vi "imp_test_v6.vi"() -> ()   [LabVIEW 2014]
uses:
  <vilib>/LabVIEW Targets/FPGA/cRIO/shared/nicrio_ModuleControls/nicrio_cRIO-9237_DataRatesRing.ctl
  <vilib>/LabVIEW Targets/FPGA/cRIO/shared/nicrio_ModuleControls/nicrio_cRIO-9237_ExcitationVoltageRing.ctl
  <vilib>/rvi/FXPMathLib/FxpSinAndCos/subVIs/nifxpmath_SinAndCos_SimConfig.ctl
  <vilib>/rvi/Emulation/niFpgaGetClockAttributes.vi
  <vilib>/rvi/Emulation/niFpgaSctlEmulationGetInTimedLoop.vi
  <vilib>/rvi/Emulation/niFpgaEmulationReportErrorSimple.vi
  <vilib>/rvi/Emulation/niFpgaProcessEmulError.vi
  <vilib>/rvi/interface/RandomDataEmulation/nirviRandomDataMultiElementFPGAFIFO.vi
  <instcachedir>/0/nirviRandomDataMultiElementFPGAFIFO_AD0CFC12EF974623A9C2E4184BC062B2.lvgen/nirviRandomDataMultiElementFPGAFIFO_AD0CFC12EF974623A9C2E4184BC062B2_025.vi
  <vilib>/rvi/interface/RandomDataEmulation/niFpgaRandomDataHandleErrors.vi
  <vilib>/rvi/Emulation/niFpgaCriticalErrorInLSC.vi
  <vilib>/rvi/eio/common/nirviEmuTemplateMethod_errors.vi
  <vilib>/rvi/FXPMathLib/FxpSinAndCos/simVIs/DllFxpSinAndCosTemp_sub.vi
  <vilib>/rvi/eio/common/nirviEmuTemplatePropertySet_errors.vi
  <vilib>/rvi/DataTransferAndStorage/Container/XNode/niFpgaContainer.xnode
  <vilib>/rvi/interface/RandomDataEmulation/nirviRandomDataFpgaMultiElementTemplate.vi
  <vilib>/eio/EIONode/EIONode.xnode
  <vilib>/rvi/FXPMathLib/FxpMul/XNode/nifxpmath_Multiplier.xnode
  <vilib>/rvi/FXPMathLib/FxpSinAndCos/XNode/nifxpmath_SinAndCos.xnode
  <vilib>/rvi/Analysis/measure/butterworth/XNode/niFpgaButterworthFilter.xnode
  <vilib>/rvi/FXPMathLib/FxpSub/XNode/nifxpmath_Sub.xnode
  <vilib>/rvi/FXPMathLib/FxpAdd/XNode/nifxpmath_Add.xnode
  <vilib>/eio/EIOPropertyNode/EIOPropertyNode.xnode
  <vilib>/rvi/eio/common/nirviEmuTemplatePropertyGet_errors.vi
  <vilib>/rvi/eio/common/nirviEmuTemplatePropertyGet_noerrors.vi
  <vilib>/rvi/eio/common/nirviEmuTemplatePropertySet_noerrors.vi
  <vilib>/rvi/FXPMathLib/sim/FxpSim.dll
panel:
  out "Strain_y (Avg2 w. f)":fxp<+/-,34,7>
  in  "Strain_y Avg2 coeff.":i32[](array[numeric])=[946630756, 63555534]
  out "Strain_y (Avg4 w. f)":fxp<+/-,35,7>
  in  "Strain_y Avg4 coeff.":i32[](array[numeric])=[946630756, 63555534]
  out "Strain_y (Avg2)":fxp<+/-,30,3>
  out "Strain_y (Avg4)":fxp<+/-,31,3>
  in  "Belt_op":fxp<+/-,7,7>
  in  "Belt_mp":fxp<+/-,6,6>
  in  "Belt_oy":fxp<+/-,7,7>
  in  "Belt_my":fxp<+/-,6,6>
  out "Fp_dc":fxp<+/-,32,10>
  out "Fy_dc":fxp<+/-,32,10>
  in  "Zero_y":bool
  in  "Zero_p":bool
  in  "mt0_omega_p":u32
  in  "Encoder reset":bool
  out "fpt_d":fxp<+/-,36,18>
  out "Dp_error_dd":fxp<+/-,36,16>
  out "Dp_error_d":fxp<+/-,33,8>
  in  "Dp_dd coeff.":i32[](array[numeric])=[946630756, 63555534]
  out "Dp_dd":fxp<+/-,36,25>
  out "dFp_PID":fxp<+/-,36,18>
  in  "dFp_PID coeff.":i32[](array[numeric])=[946630756, 63555534]
  out "fpt_i":fxp<+/-,34,18>
  in  "Bv_p":fxp<+/-,22,8>
  in  "Kv_p":fxp<+/-,22,8>
  out "Dp_error":fxp<+/-,22,7>
  out "Dpr_sin":fxp<+/-,22,7>
  in  "Sin offset_p":fxp<+/-,22,7>
  in  "Sin magnitude_p":fxp<+/-,21,6>
  out "Dpr_sin_dd":fxp<+/-,35,20>
  out "Dpr_sin_d":fxp<+/-,33,15>
  out "Sin omega_p":fxp<+/-,34,9>
  in  "Sin wave freq._p (Hz)":fxp<+/-,32,6>
  in  "Dpr_step":fxp<+/-,22,7>
  out "Dpr_for":fxp<+/-,22,7>
  in  "Command_p":i16(ring) items=["Step", "Sine"]
  in  "Ki_p":fxp<+/-,36,9>
  out "Fp_PID":fxp<+/-,36,16>
  in  "fp_tolorance":fxp<+,22,6>
  out "fp_tilde":fxp<+/-,33,10>
  in  "Kd_p":fxp<+/-,36,9>
  in  "Kp_p":fxp<+/-,36,9>
  out "Fr_p":fxp<+/-,32,10>
  in  "S/F coeff_p":fxp<+/-,25,-10>
  in  "S/F coeff_y":fxp<+/-,25,-10>
  out "va_p":fxp<+/-,36,7>
  out "vb_p":fxp<+/-,37,8>
  out "vq_p_F":fxp<+/-,20,5> format="%.57g"
  out "vd_p_F":fxp<+/-,20,5>
  in  "dFp_add":bool
  in  "Stop motor_p":bool
  out "Force_p":fxp<+/-,32,10>
  in  "Strain selection_p":i16(ring) items=["Raw", "Avg.8", "Avg.8 w. filter"]
  out "Strain_p (Avg8 w. f)":fxp<+/-,36,8>
  in  "Strain_p Avg.8 coeff.":i32[](array[numeric])=[946630756, 63555534]
  out "Strain_p (Avg8)":fxp<+/-,36,4>
  out "Raw Strain_p":fxp<+/-,36,4>
  out "Mod6/AI3":fxp<+/-,36,4>
  in  "Strain gage reset_p":bool
  out "Dp_d (mm/s)":fxp<+/-,36,11>
  out "omega_p (rad/s)":fxp<+/-,20,9>
  out "mt_omega_p":u32
  out "rad_p(NrTheta)":fxp<+/-,33,20>
  out "D_p(mm)":fxp<+/-,32,7>
  out "Encoder Position_p":i32
  in  "Encoder reset_p":bool
  out "Strain_y (Avg8 w. f)":fxp<+/-,36,8>
  in  "Strain_y Avg8 coeff.":i32[](array[numeric])=[-898916953, 1957103773, 3888751]
  out "Dyr_for":fxp<+/-,22,7>
  in  "Command_y":i16(ring) items=["Step", "Sine"]
  out "Strain_y (Avg8)":fxp<+/-,36,4>
  in  "Strain selection_y":i16(ring) items=["Raw", "Avg.8", "Avg.8 w. filter", "Avg.4", "Avg.4 w. filter", "Avg.2", "Avg.2 w. filter"]
  out "vb_y":fxp<+/-,38,8>
  out "va_y":fxp<+/-,38,8>
  out "fyt_d":fxp<+/-,36,18>
  out "Fr_y":fxp<+/-,32,10>
  in  "Bv_y":fxp<+/-,22,8>
  out "Dy_error_dd":fxp<+/-,36,16>
  out "Dy_error_d":fxp<+/-,33,8>
  in  "Kv_y":fxp<+/-,22,8>
  out "Dy_error":fxp<+/-,22,7>
  out "Dyr_sin_dd":fxp<+/-,35,20>
  out "Dyr_sin_d":fxp<+/-,33,15>
  out "Sin omega_y":fxp<+/-,34,9>
  out "Dyr_sin":fxp<+/-,22,7>
  in  "Sin offset_y":fxp<+/-,22,7>
  in  "Sin magnitude_y":fxp<+/-,21,6>
  out "Time now(s)":fxp<+,52,14>
  in  "Sin wave freq._y (Hz)":fxp<+/-,32,6>
  in  "Dyr_step":fxp<+/-,22,7>
  in  "Drive mode":i16(ring) items=["Backward", "Forward"]
  out "Dy_dd":fxp<+/-,36,25>
  in  "Dy_dd coeff.":i32[](array[numeric])=[946630756, 63555534]
  out "dFy_PID":fxp<+/-,36,18>
  in  "dFy_PID coeff.":i32[](array[numeric])=[946630756, 63555534]
  out "fyt_i":fxp<+/-,36,16>
  out "Fy_PID":fxp<+/-,36,16>
  in  "fy_tolorance":fxp<+,22,6>
  in  "Ki_y":fxp<+/-,36,9>
  in  "Kd_y":fxp<+/-,36,9>
  out "fy_tilde":fxp<+/-,32,10>
  in  "Kp_y":fxp<+/-,36,9>
  out "vq_y_F":fxp<+/-,20,5> format="%.57g"
  out "vd_y_F":fxp<+/-,20,5>
  in  "dFy_add":bool
  in  "Stop motor_y":bool
  out "Dy_d (mm/s)":fxp<+/-,36,11>
  out "omega_y (rad/s)":fxp<+/-,20,9>
  in  "mt0_omega_y":u32
  out "mt_omega_y":u32
  out "rad_y(NrTheta)":fxp<+/-,33,20>
  out "D_y(mm)":fxp<+/-,32,7>
  out "Encoder Position_y":i32
  in  "Encoder reset_y":bool
  in  "Ini coe.":bool
  out "Loop rate (kHz)":fxp<+/-,36,7>
  out "Force_y":fxp<+/-,32,10>
  out "Raw Strain_y":fxp<+/-,36,4>
  in  "Strain gage reset_y":bool
  in  "Stop (Strain)":bool
  out "Mod6/AI2":fxp<+/-,36,4>
  in  "Excitation Voltage":T1 items=["2.5 Volts", "3.3 Volts", "5.0 Volts", "10.0 Volts", "External Excitation"]
  in  "Data Rate":T2=1 items=["50.000 kS/s (NI 9237)"=1, "25.000 kS/s (NI 9237)"=2, "16.667 kS/s (NI 9237)"=3, "12.500 kS/s (NI 9237)"=4, "10.000 kS/s (NI 9237)"=5, "8.333 kS/s (NI 9237)"=6, "7.143 kS/s (NI 9237)"=7, "6.250 kS/s (NI 9237)"=8, "5.556 kS/s (NI 9237)"=9, "5.000 kS/s (NI 9237)"=10, "4.545 kS/s (NI 9237)"=11, "4.167 kS/s (NI 9237)"=12, "3.846 kS/s (NI 9237)"=13, "3.571 kS/s (NI 9237)"=14, "3.333 kS/s (NI 9237)"=15, "3.125 kS/s (NI 9237)"=16, "2.941 kS/s (NI 9237)"=17, "2.778 kS/s (NI 9237)"=18, "2.632 kS/s (NI 9237)"=19, "2.500 kS/s (NI 9237)"=20, "2.381 kS/s (NI 9237)"=21, "2.273 kS/s (NI 9237)"=22, "2.174 kS/s (NI 9237)"=23, "2.083 kS/s (NI 9237)"=24, "2.000 kS/s (NI 9237)"=25, "1.923 kS/s (NI 9237)"=26, "1.852 kS/s (NI 9237)"=27, "1.786 kS/s (NI 9237)"=28, "1.724 kS/s (NI 9237)"=29, "1.667 kS/s (NI 9237)"=30, "1.613 kS/s (NI 9237)"=31]
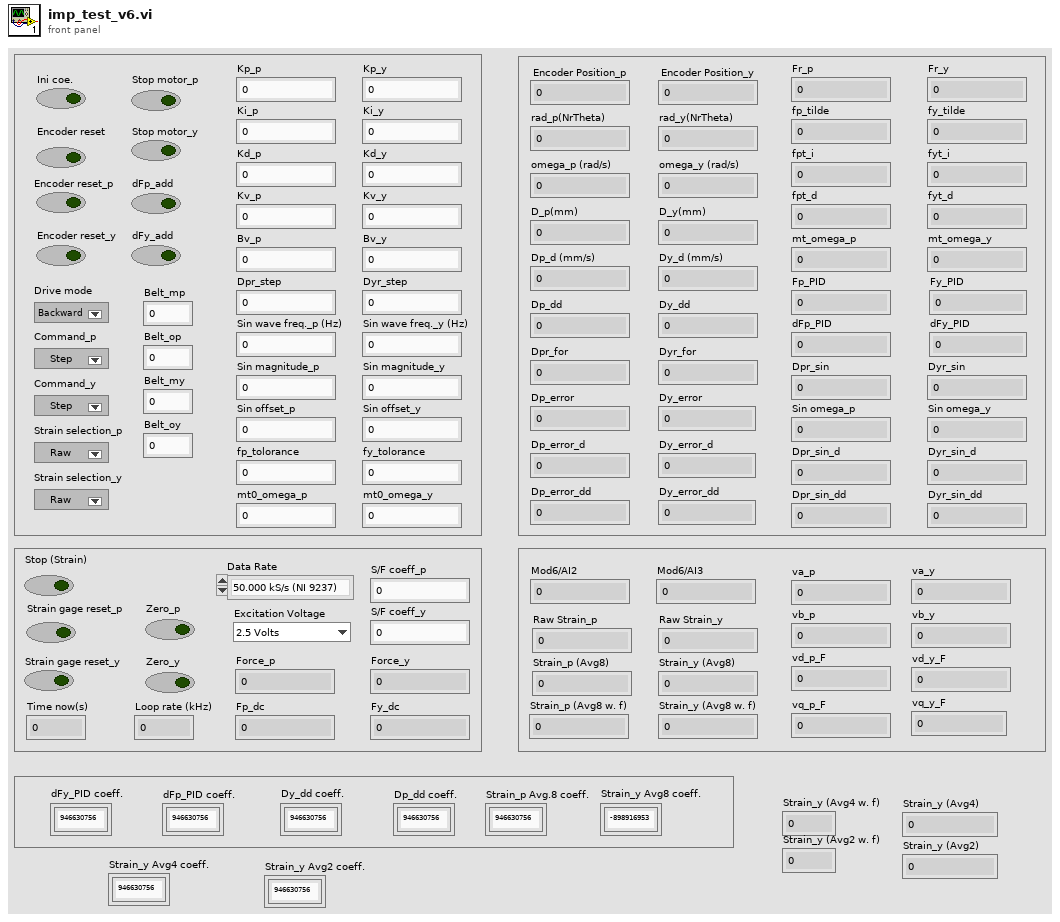
[diagram p1: front panel]
types:
  T1 = typedef "nicrio_cRIO-9237_ExcitationVoltageRing.ctl" = u8
  T2 = typedef "nicrio_cRIO-9237_DataRatesRing.ctl" = u8
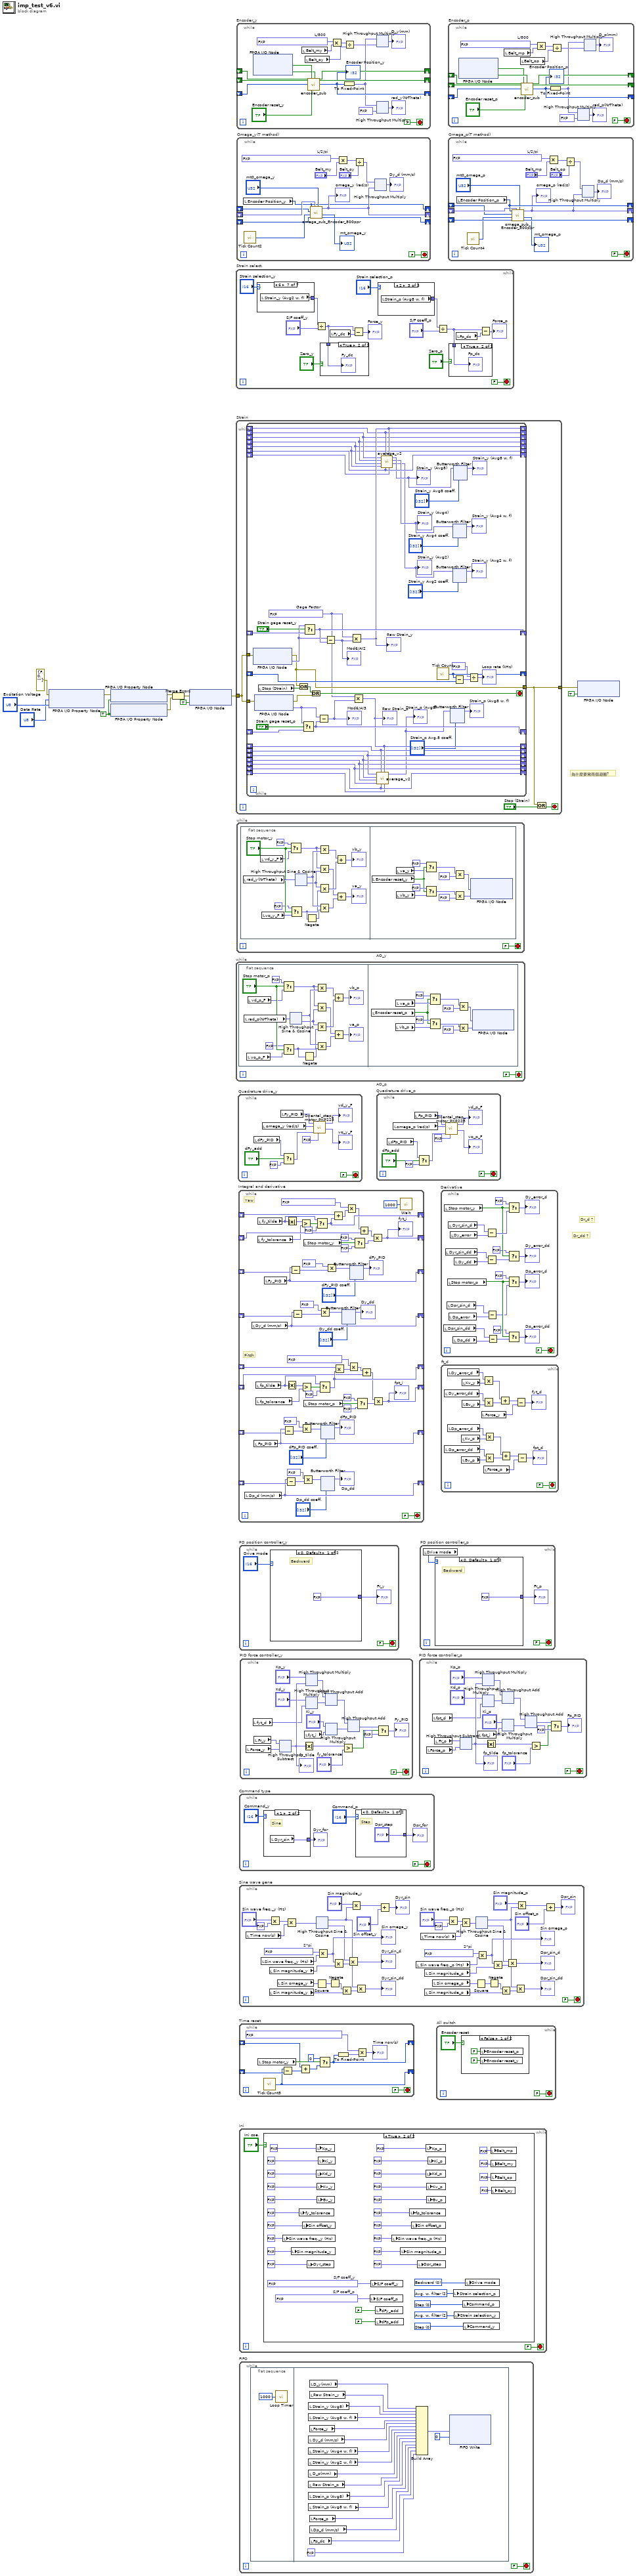
[diagram p0: block diagram]
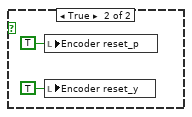
[diagram p2: hidden frame]
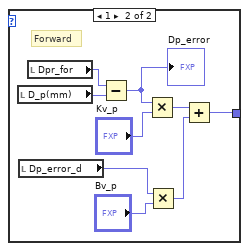
[diagram p3: hidden frame]
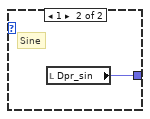
[diagram p4: hidden frame]
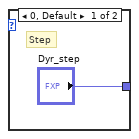
[diagram p5: hidden frame]
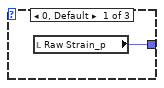
[diagram p8: hidden frame]
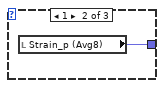
[diagram p9: hidden frame]
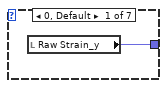
[diagram p10: hidden frame]
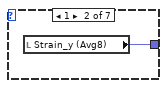
[diagram p11: hidden frame]
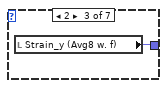
[diagram p12: hidden frame]
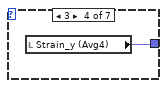
[diagram p13: hidden frame]
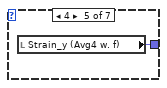
[diagram p14: hidden frame]
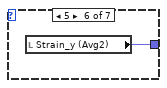
[diagram p15: hidden frame]
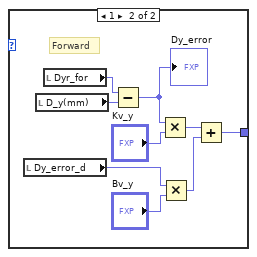
[diagram p16: hidden frame]
diagram:
  w5 = TRUE ("Half-Bridge Enable")
  # "為什麼要寫兩個迴圈?"
  # "Dr_dd ?"
  # "Dr_d ?"
  n1 = xnode "FPGA I/O Property Node"("error in"=errorcluster {"status"=FALSE, "code"=0, "source"=""}, "Data Rate"="Data Rate", "Excitation Voltage"="Excitation Voltage") -> ("error out"=w10:errorcluster)  [unwired: 1 in, 1 out]
  n2 = xnode "FPGA I/O Property Node"("error in"=w10, "Half-Bridge Enable"=w5) -> ("error out"=w3:errorcluster)  [unwired: 1 in, 1 out]
  n3 = xnode "FPGA I/O Property Node"("Half-Bridge Enable"=w5) -> ("error out"=w2:errorcluster)  [unwired: 2 in, 1 out]
  n4 = Merge Errors(w3, w2) -> (w4:errorcluster)
  n5 = xnode "FPGA I/O Node"("error in"=w4, "Mod6/Start"=TRUE) -> ("error out"=w8:errorcluster)  [unwired: 1 in, 1 out]
  n6 = while "Strain select." {
    stop <- FALSE stop-if-true
    n7 = case shown="6" "Strain selection_y" {
      tunnel: [w33 w34 w35 w36 w37 w38 w39] -> w26
      frame 0, Default {
        n8 = local read "Raw Strain_y"() -> (w33:fxp<+/-,36,4>)
      }
      frame 1 {
        n9 = local read "Strain_y (Avg8)"() -> (w34:fxp<+/-,36,4>)
      }
      frame 2 {
        n10 = local read "Strain_y (Avg8 w. f)"() -> (w35:fxp<+/-,36,8>)
      }
      frame 3 {
        n11 = local read "Strain_y (Avg4)"() -> (w36:fxp<+/-,31,3>)
      }
      frame 4 {
        n12 = local read "Strain_y (Avg4 w. f)"() -> (w37:fxp<+/-,35,7>)
      }
      frame 5 {
        n13 = local read "Strain_y (Avg2)"() -> (w38:fxp<+/-,30,3>)
      }
      frame 6 {
        n14 = local read "Strain_y (Avg2 w. f)"() -> (w39:fxp<+/-,34,7>)
      }
    }
    n15 = Divide(x=w26, y="S/F coeff_y") -> (x/y=w19:fxp<+/-,32,10>)
    n16 = case shown="True" "Zero_y" {
      tunnel: w19 -> [_ w29]
      frame False {
      }
      frame True {
        "Fy_dc" <- w29
      }
    }
    n17 = local read "Fy_dc"() -> (w20:fxp<+/-,32,10>)
    n18 = Subtract(x=w19, y=w20) -> (x-y=→"Force_y":fxp<+/-,33,11>)
    n19 = case shown="2" "Strain selection_p" {
      tunnel: [w30 w31 w32] -> w24
      frame 0, Default {
        n20 = local read "Raw Strain_p"() -> (w30:fxp<+/-,36,4>)
      }
      frame 1 {
        n21 = local read "Strain_p (Avg8)"() -> (w31:fxp<+/-,36,4>)
      }
      frame 2 {
        n22 = local read "Strain_p (Avg8 w. f)"() -> (w32:fxp<+/-,36,8>)
      }
    }
    n23 = Divide(x=w24, y="S/F coeff_p") -> (x/y=w16:fxp<+/-,32,10>)
    n24 = case shown="True" "Zero_p" {
      tunnel: w16 -> [_ w28]
      frame False {
      }
      frame True {
        "Fp_dc" <- w28
      }
    }
    n25 = local read "Fp_dc"() -> (w14:fxp<+/-,32,10>)
    n26 = Subtract(x=w16, y=w14) -> (x-y=→"Force_p":fxp<+/-,33,11>)
  }
  n27 = while "Strain" {
    tunnel: w8 -> [w42]
    tunnel: [w40] -> w1
    stop <- w41 stop-if-true
    n28 = while {
      tunnel: w42 -> [w94]
      tunnel: [w67] -> w40
      shift-right: [w91] -> _
      shift-left: _ -> [w92]
      shift-right: [w87] -> _
      shift-left: _ -> [w88]
      shift-right: [w82] -> _
      shift-left: _ -> [w81]
      shift-right: [w81] -> _
      shift-left: _ -> [w80]
      shift-right: [w80] -> _
      shift-left: _ -> [w79]
      shift-right: [w79] -> _
      shift-left: _ -> [w78]
      shift-right: [w78] -> _
      shift-left: _ -> [w77]
      shift-right: [w77] -> _
      shift-left: _ -> [w76]
      shift-right: [w76] -> _
      shift-left: _ -> [w75]
      tunnel: w42 -> [w71]
      shift-right: [w64] -> _
      shift-left: _ -> [w65]
      shift-right: [w60] -> _
      shift-left: _ -> [w59]
      shift-right: [w59] -> _
      shift-left: _ -> [w58]
      shift-right: [w58] -> _
      shift-left: _ -> [w57]
      shift-right: [w57] -> _
      shift-left: _ -> [w56]
      shift-right: [w56] -> _
      shift-left: _ -> [w55]
      shift-right: [w55] -> _
      shift-left: _ -> [w54]
      shift-right: [w54] -> _
      shift-left: _ -> [w53]
      stop <- w68 stop-if-true
      w62 = fxp<+,20,2> 2.115001678466797  # Gage Factor
      n29 = xnode "FPGA I/O Node"("error in"=w94) -> ("error out"=w67:errorcluster, "Mod6/AI2"=w89:fxp<+/-,24,-4>)  [unwired: 1 in, 1 out]
      n30 = xnode "FPGA I/O Node"("error in"=w71) -> ("error out"=w69:errorcluster, "Mod6/AI3"=w63:fxp<+/-,24,-4>)  [unwired: 1 in, 1 out]
      n31 = local read "Stop (Strain)"() -> (w93:bool)
      n32 = Or(x=w67, y=w93) -> (x .or. y?=w70:bool)
      n33 = Select(t=w63, s="Strain gage reset_p", f=w65) -> (s? t:f=w64:fxp<+/-,24,-4>)
      n34 = Select(t=w89, s="Strain gage reset_y", f=w92) -> (s? t:f=w91:fxp<+/-,24,-4>)
      n35 = Or(x=w70, y=w69) -> (x .or. y?=w68:bool)
      n36 = Subtract(x=w63, y=w64) -> (x-y=w61:fxp<+/-,30,-3>)
      "Mod6/AI3" <- w61
      n37 = Subtract(x=w89, y=w91) -> (x-y=w90:fxp<+/-,30,-3>)
      "Mod6/AI2" <- w90
      n38 = Multiply(x=w62, y=w90) -> (x*y=w82:fxp<+/-,41,6>)
      "Raw Strain_y" <- w82
      n39 = Multiply(x=w62, y=w61) -> (x*y=w60:fxp<+/-,50,-1>)
      "Raw Strain_p" <- w60
      n40 = call "average_v2.vi"("Numeric 8"=w53, "Numeric"=w60, "Numeric 7"=w54, "Numeric 2"=w59, "Numeric 6"=w55, "Numeric 5"=w56, "Numeric 4"=w57, "Numeric 3"=w58) -> ("Mean (8pt)"=w52:fxp<+/-,32,4>)  [unwired: 1 in, 2 out]
      "Strain_p (Avg8)" <- w52
      n41 = call "average_v2.vi"("Numeric 8"=w75, "Numeric"=w82, "Numeric 7"=w76, "Numeric 2"=w81, "Numeric 6"=w77, "Numeric 5"=w78, "Numeric 4"=w79, "Numeric 3"=w80) -> ("Mean (2pt)"=w46:fxp<+/-,30,3>, "Mean (4pt)"=w49:fxp<+/-,31,3>, "Mean (8pt)"=w74:fxp<+/-,32,4>)  [unwired: 1 in]
      "Strain_y (Avg8)" <- w74
      "Strain_y (Avg4)" <- w49
      "Strain_y (Avg2)" <- w46
      n42 = call "Tick Count"() -> ("Tick Count(uSec)"=w87:u32)
      n43 = xnode "Butterworth Filter"("input data"=w52, "scaled coefficients"="Strain_p Avg.8 coeff.") -> ("output data"=→"Strain_p (Avg8 w. f)":fxp<+/-,36,8>)  [unwired: 1 in]
      n44 = xnode "Butterworth Filter"("input data"=w49, "scaled coefficients"="Strain_y Avg4 coeff.") -> ("output data"=→"Strain_y (Avg4 w. f)":fxp<+/-,35,7>)  [unwired: 1 in]
      n45 = xnode "Butterworth Filter"("input data"=w46, "scaled coefficients"="Strain_y Avg2 coeff.") -> ("output data"=→"Strain_y (Avg2 w. f)":fxp<+/-,34,7>)  [unwired: 1 in]
      n46 = xnode "Butterworth Filter"("input data"=w74, "scaled coefficients"="Strain_y Avg8 coeff.") -> ("output data"=→"Strain_y (Avg8 w. f)":fxp<+/-,32,4>)  [unwired: 1 in]
      n47 = Subtract(x=w87, y=w88) -> (x-y=w85:fxp<+/-,32,16>)
      n48 = Divide(x=fxp<+,7,10> 1000.0, y=w85) -> (x/y=→"Loop rate (kHz)":fxp<+/-,40,27>)
    }
    n49 = Or(x=w40, y="Stop (Strain)") -> (x .or. y?=w41:bool)
  }
  n50 = while "AO_p" {
    stop <- FALSE stop-if-true
    n51 = flat-sequence {
      frame #0 {
        n52 = local read "rad_p(NrTheta)"() -> (w139:fxp<+/-,33,20>)
        n53 = local read "vq_p_F"() -> (w140:fxp<+/-,20,5>)
        n54 = local read "vd_p_F"() -> (w142:fxp<+/-,20,5>)
        n55 = Select(t=fxp<+/-,20,5> 0.0, s="Stop motor_p", f=w142) -> (s? t:f=w131:fxp<+/-,20,5>)
        n56 = Select(t=fxp<+,1,1> 0.0, s="Stop motor_p", f=w140) -> (s? t:f=w130:fxp<+/-,20,5>)
        n57 = xnode "High Throughput Sine & Cosine"("x (pi)"=w139) -> ("sin(x)"=w133:fxp<+/-,16,2>, "cos(x)"=w132:fxp<+/-,16,2>)
        n58 = Negate(x=w130) -> (-x=w138:fxp<+/-,21,6>)
        n59 = Multiply(x=w131, y=w133) -> (x*y=w137:fxp<+/-,36,7>)
        n60 = Multiply(x=w131, y=w132) -> (x*y=w135:fxp<+/-,36,7>)
        n61 = Multiply(x=w132, y=w130) -> (x*y=w136:fxp<+/-,36,7>)
        n62 = Multiply(x=w133, y=w138) -> (x*y=w134:fxp<+/-,35,6>)
        n63 = Add(x=w137, y=w136) -> (x+y=→"vb_p":fxp<+/-,37,8>)
        n64 = Add(x=w135, y=w134) -> (x+y=→"va_p":fxp<+/-,36,7>)
      }
      frame #1 {
        n65 = local read "Encoder reset_p"() -> (w175:bool)
        n66 = local read "vb_p"() -> (w176:fxp<+/-,37,8>)
        n67 = local read "va_p"() -> (w177:fxp<+/-,36,7>)
        n68 = Select(t=fxp<+,2,2> 3.0, s=w175, f=w177) -> (s? t:f=w183:fxp<+/-,36,7>)
        n69 = Select(t=fxp<+,1,1> 0.0, s=w175, f=w176) -> (s? t:f=w182:fxp<+/-,37,8>)
        n70 = Multiply(x=w183, y=fxp<+/-,1,0> -0.5) -> (x*y=w178:fxp<+/-,36,6>)
        n71 = Multiply(x=w182, y=fxp<+/-,1,0> -0.5) -> (x*y=w179:fxp<+/-,36,6>)
        n72 = xnode "FPGA I/O Node"("Mod8/AO0"=w178, "Mod8/AO1"=w179) -> ()  [unwired: 2 in, 2 out]
      }
    }
  }
  n73 = while "Encoder_y" {
    shift-right: [w201] -> _
    shift-left: _ -> [w202]
    shift-right: [w203] -> _
    shift-left: _ -> [w204]
    shift-right: [w196] -> _
    shift-left: _ -> [w200]
    stop <- FALSE stop-if-true
    w190 = fxp<+/-,20,-5> 0.002499997615814209  # L/800
    n74 = xnode "FPGA I/O Node"() -> ("Mod4/DI3"=w199:bool, "Mod4/DI4"=w198:bool)  [unwired: 2 in, 2 out]
    n75 = local read "Belt_my"() -> (w189:fxp<+/-,6,6>)
    n76 = local read "Belt_oy"() -> (w187:fxp<+/-,7,7>)
    n77 = call "encoder_sub.vi"("A_pre"=w202, "B_pre"=w204, "Encoder Position_pre"=w200, "A input"=w199, "Encoder Position Reset"="Encoder reset_y", "B input"=w198) -> ("A"=w201:bool, "B"=w203:bool, "Encoder Position (Counts)"=w196:i32)  [unwired: 19 in]
    "Encoder Position_y" <- w196
    n78 = Multiply(x=w190, y=w189) -> (x*y=w188:fxp<+/-,26,1>)
    n79 = To Fixed-Point(number=w196) -> (fixed-point=w195:fxp<+/-,32,32>)  [unwired: 1 in]
    n80 = Divide(x=w188, y=w187) -> (x/y=w186:fxp<+/-,33,1>)
    n81 = xnode ("High Throughput Multiply")("x"=w195, "y"=w186) -> ("x*y"=→"D_y(mm)":fxp<+/-,64,33>)
    n82 = xnode ("High Throughput Multiply")("x"=w195, "y"=fxp<+/-,16,1> 0.125) -> ("x*y"=→"rad_y(NrTheta)":fxp<+/-,48,33>)
  }
  n83 = while "AO_y" {
    stop <- FALSE stop-if-true
    n84 = flat-sequence {
      frame #0 {
        n85 = local read "rad_y(NrTheta)"() -> (w222:fxp<+/-,33,20>)
        n86 = local read "vd_y_F"() -> (w220:fxp<+/-,20,5>)
        n87 = local read "vq_y_F"() -> (w219:fxp<+/-,20,5>)
        n88 = Select(t=fxp<+/-,20,5> 0.0, s="Stop motor_y", f=w220) -> (s? t:f=w214:fxp<+/-,20,5>)
        n89 = Select(t=fxp<+/-,20,5> 0.0, s="Stop motor_y", f=w219) -> (s? t:f=w213:fxp<+/-,20,5>)
        n90 = xnode "High Throughput Sine & Cosine"("x (pi)"=w222) -> ("sin(x)"=w216:fxp<+/-,17,2>, "cos(x)"=w215:fxp<+/-,17,2>)
        n91 = Negate(x=w213) -> (-x=w212:fxp<+/-,21,6>)
        n92 = Multiply(x=w214, y=w216) -> (x*y=w211:fxp<+/-,37,7>)
        n93 = Multiply(x=w214, y=w215) -> (x*y=w209:fxp<+/-,37,7>)
        n94 = Multiply(x=w215, y=w213) -> (x*y=w210:fxp<+/-,37,7>)
        n95 = Multiply(x=w216, y=w212) -> (x*y=w208:fxp<+/-,36,6>)
        n96 = Add(x=w211, y=w210) -> (x+y=→"vb_y":fxp<+/-,38,8>)
        n97 = Add(x=w209, y=w208) -> (x+y=→"va_y":fxp<+/-,37,7>)
      }
      frame #1 {
        n98 = local read "Encoder reset_y"() -> (w255:bool)
        n99 = local read "va_y"() -> (w254:fxp<+/-,38,8>)
        n100 = local read "vb_y"() -> (w253:fxp<+/-,38,8>)
        n101 = Select(t=fxp<+,2,2> 3.0, s=w255, f=w254) -> (s? t:f=w259:fxp<+/-,38,8>)
        n102 = Select(t=fxp<+,1,1> 0.0, s=w255, f=w253) -> (s? t:f=w258:fxp<+/-,38,8>)
        n103 = Multiply(x=w259, y=fxp<+/-,1,0> -0.5) -> (x*y=w262:fxp<+/-,39,8>)
        n104 = Multiply(x=w258, y=fxp<+/-,1,0> -0.5) -> (x*y=w263:fxp<+/-,37,6>)
        n105 = xnode "FPGA I/O Node"("Mod8/AO2"=w262, "Mod8/AO3"=w263) -> ()  [unwired: 2 in, 2 out]
      }
    }
  }
  n106 = while "Omega_y(T method)" {
    shift-right: [w270] -> _
    shift-left: _ -> [w271]
    shift-right: [w273] -> _
    shift-left: _ -> [w275]
    shift-right: [w277] -> _
    shift-left: _ -> [w278]
    stop <- FALSE stop-if-true
    w268 = fxp<+/-,32,0> 0.3183098859153688  # L/2/pi
    n107 = local read "Encoder Position_y"() -> (w270:i32)
    n108 = call "Tick Count2"() -> ("Tick Count(Ticks)"=w279:u32)
    n109 = call "omega_sub_Encoder_800ppr.vi"("mt0"="mt0_omega_y", "omega_pre"=w275, "ticks_m_pre"=w278, "ticks"=w279, "count_pre"=w271, "count"=w270) -> ("ticks_m"=w277:u32, "mt"=→"mt_omega_y":u32, "omega"=w273:fxp<+/-,20,9>)  [unwired: 3 in]
    "omega_y (rad/s)" <- w273
    n110 = Multiply(x=w268, y="Belt_my") -> (x*y=w266:fxp<+/-,38,6>)
    n111 = Divide(x=w266, y="Belt_oy") -> (x/y=w264:fxp<+/-,20,1>)
    n112 = xnode ("High Throughput Multiply")("x"=w264, "y"=w273) -> ("x*y"=→"Dy_d (mm/s)":fxp<+/-,40,10>)
  }
  n113 = while "Quadrature drive_y" {
    stop <- FALSE stop-if-true
    n114 = local read "dFy_PID"() -> (w281:fxp<+/-,36,18>)
    n115 = local read "omega_y (rad/s)"() -> (w289:fxp<+/-,20,9>)
    n116 = local read "Fy_PID"() -> (w282:fxp<+/-,36,16>)
    n117 = Select(t=w281, s="dFy_add", f=fxp<+,1,1> 0.0) -> (s? t:f=w285:fxp<+/-,36,18>)
    n118 = call "Oriental_step_motor_PKP225.vi"("F_Threshold"=fxp<+,12,12> 10.0, "dFmr"=w285, "omega"=w289, "Fmr"=w282) -> ("vq_F"=→"vq_y_F":fxp<+/-,20,5>, "vd_F"=→"vd_y_F":fxp<+/-,20,5>)  [unwired: 6 in]
  }
  n119 = while "Integral and derivative" {
    shift-right: [w345] -> _
    shift-left: _ -> [w344]
    shift-right: [w337] -> _
    shift-left: _ -> [w336]
    shift-right: [w347] -> _
    shift-left: _ -> [w348]
    shift-right: [w327] -> _
    shift-left: _ -> [w326]
    shift-right: [w313] -> _
    shift-left: _ -> [w316]
    shift-right: [w306] -> _
    shift-left: _ -> [w305]
    shift-right: [w300] -> _
    shift-left: _ -> [w299]
    shift-right: [w295] -> _
    shift-left: _ -> [w296]
    stop <- FALSE stop-if-true
    # "Pitch"
    # "Yaw"
    n120 = local read "Dp_d (mm/s)"() -> (w295:fxp<+/-,36,11>)
    n121 = local read "Dy_d (mm/s)"() -> (w327:fxp<+/-,36,11>)
    n122 = local read "Fp_PID"() -> (w300:fxp<+/-,36,16>)
    n123 = local read "fp_tilde"() -> (w317:fxp<+/-,33,10>)
    n124 = local read "fp_tolorance"() -> (w320:fxp<+,22,6>)
    n125 = local read "fy_tolorance"() -> (w323:fxp<+,22,6>)
    n126 = local read "fy_tilde"() -> (w349:fxp<+/-,32,10>)
    n127 = local read "Fy_PID"() -> (w347:fxp<+/-,36,16>)
    n128 = Subtract(x=w300, y=w299) -> (x-y=w304:fxp<+/-,37,17>)
    n129 = Subtract(x=w295, y=w296) -> (x-y=w297:fxp<+/-,37,12>)
    n130 = Absolute Value(x=w317) -> (abs(x)=w321:fxp<+,33,10>)
    n131 = Absolute Value(x=w349) -> (abs(x)=w351:fxp<+,32,10>)
    n132 = Subtract(x=w347, y=w348) -> (x-y=w335:fxp<+/-,37,17>)
    n133 = Subtract(x=w327, y=w326) -> (x-y=w329:fxp<+/-,36,11>)
    n134 = Greater?(x=w351, y=w323) -> (0:w352:bool)
    n135 = Greater?(x=w321, y=w320) -> (0:w319:bool)
    n136 = Multiply(x=fxp<+,7,10> 1000.0, y=w304) -> (x*y=w302:fxp<+/-,32,18>)
    n137 = Multiply(x=fxp<+,7,10> 1000.0, y=w297) -> (x*y=w293:fxp<+/-,36,21>)
    n138 = local read "Stop motor_y"() -> (w338:bool)
    n139 = local read "Stop motor_p"() -> (w308:bool)
    n140 = Select(t=w349, s=w352, f=fxp<+/-,33,11> 0.0) -> (s? t:f=w345:fxp<+/-,33,11>)
    n141 = Select(t=w317, s=w319, f=fxp<+,1,1> 0.0) -> (s? t:f=w313:fxp<+/-,33,10>)
    n142 = Multiply(x=fxp<+,7,10> 1000.0, y=w329) -> (x*y=w328:fxp<+/-,36,21>)
    n143 = xnode "Butterworth Filter"("input data"=w302, "scaled coefficients"="dFp_PID coeff.") -> ("output data"=→"dFp_PID":fxp<+/-,36,22>)  [unwired: 1 in]
    n144 = xnode "Butterworth Filter"("input data"=w293, "scaled coefficients"="Dp_dd coeff.") -> ("output data"=→"Dp_dd":fxp<+/-,36,25>)  [unwired: 1 in]
    n145 = Multiply(x=fxp<+,7,10> 1000.0, y=w335) -> (x*y=w332:fxp<+/-,32,18>)
    n146 = Add(x=w344, y=w345) -> (x+y=w350:fxp<+/-,34,12>)
    n147 = Multiply(x=w316, y=w313) -> (x*y=w315:fxp<+/-,34,12>)
    n148 = xnode "Butterworth Filter"("input data"=w328, "scaled coefficients"="Dy_dd coeff.") -> ("output data"=→"Dy_dd":fxp<+/-,36,25>)  [unwired: 1 in]
    n149 = Multiply(x=fxp<+/-,30,12> 0.000499725341796875, y=w350) -> (x*y=w343:fxp<+/-,34,10>)
    n150 = Multiply(x=fxp<+/-,30,12> 0.000499725341796875, y=w315) -> (x*y=w312:fxp<+/-,34,10>)
    n151 = xnode "Butterworth Filter"("input data"=w332, "scaled coefficients"="dFy_PID coeff.") -> ("output data"=→"dFy_PID":fxp<+/-,36,22>)  [unwired: 1 in]
    n152 = Select(t=fxp<+,1,1> 0.0, s=w338, f=fxp<+,1,1> 1.0) -> (s? t:f=w341:fxp<+,1,1>)
    n153 = Select(t=fxp<+,1,1> 0.0, s=w308, f=fxp<+,1,1> 1.0) -> (s? t:f=w310:fxp<+,1,1>)
    n154 = Add(x=w343, y=w336) -> (x+y=w342:fxp<+/-,36,16>)
    n155 = Add(x=w312, y=w305) -> (x+y=w311:fxp<+/-,36,16>)
    n156 = Multiply(x=w342, y=w341) -> (x*y=w337:fxp<+/-,34,18>)
    "fyt_i" <- w337
    n157 = Multiply(x=w311, y=w310) -> (x*y=w306:fxp<+/-,34,18>)
    "fpt_i" <- w306
    n158 = call "Wait"("Count(uSec)"=u32 1000) -> ()  [unwired: 1 out]
  }
  n159 = while "PD position controller_y" {
    stop <- FALSE stop-if-true
    n160 = case shown="0, Default" "Drive mode" {
      tunnel: [fxp<+/-,62,19> 0.0 w391] -> w387
      frame 0, Default {
        # "Backward"
      }
      frame 1 {
        # "Forward"
        n161 = local read "Dy_error_d"() -> (w393:fxp<+/-,33,8>)
        n162 = local read "D_y(mm)"() -> (w398:fxp<+/-,32,7>)
        n163 = local read "Dyr_for"() -> (w390:fxp<+/-,22,7>)
        n164 = Subtract(x=w390, y=w398) -> (x-y=w397:fxp<+/-,33,8>)
        "Dy_error" <- w397
        n165 = Multiply(x=w397, y="Kv_y") -> (x*y=w395:fxp<+/-,54,15>)
        n166 = Multiply(x=w393, y="Bv_y") -> (x*y=w392:fxp<+/-,55,16>)
        n167 = Add(x=w395, y=w392) -> (x+y=w391:fxp<+/-,55,16>)
      }
    }
    "Fr_y" <- w387
  }
  n168 = while "Command type" {
    stop <- FALSE stop-if-true
    n169 = case shown="1" "Command_y" {
      tunnel: ["Dyr_step" w407] -> w402
      frame 0, Default {
        # "Step"
      }
      frame 1 {
        # "Sine"
        n170 = local read "Dyr_sin"() -> (w407:fxp<+/-,22,7>)
      }
    }
    "Dyr_for" <- w402
    n171 = case shown="0, Default" "Command_p" {
      tunnel: ["Dpr_step" w405] -> w400
      frame 0, Default {
        # "Step"
      }
      frame 1 {
        # "Sine"
        n172 = local read "Dpr_sin"() -> (w405:fxp<+/-,22,7>)
      }
    }
    "Dpr_for" <- w400
  }
  n173 = while "Sine wave gene" {
    stop <- FALSE stop-if-true
    w413 = fxp<+,20,3> 6.2831878662109375  # 2*pi
    w445 = fxp<+,20,3> 6.2831878662109375  # 2*pi
    n174 = local read "Time now(s)"() -> (w451:fxp<+,52,14>)
    n175 = local read "Sin wave freq._y (Hz)"() -> (w444:fxp<+/-,32,6>)
    n176 = Multiply(x="Sin wave freq._y (Hz)", y=fxp<+/-,10,3> 2.0) -> (x*y=w452:fxp<+/-,41,9>)
    n177 = local read "Sin magnitude_y"() -> (w442:fxp<+/-,21,6>)
    n178 = local read "Sin magnitude_y"() -> (w435:fxp<+/-,21,6>)
    n179 = local read "Sin omega_y"() -> (w438:fxp<+/-,34,9>)
    n180 = Multiply(x=w452, y=w451) -> (x*y=w450:fxp<+/-,41,19>)
    n181 = Square(x=w438) -> (x^2=w437:fxp<+,34,18>)
    n182 = xnode "High Throughput Sine & Cosine"("x (pi)"=w450) -> ("sin(x)"=w432:fxp<+/-,16,2>, "cos(x)"=w440:fxp<+/-,16,2>)
    n183 = Multiply(x=w445, y=w444) -> (x*y=w443:fxp<+/-,34,9>)
    "Sin omega_y" <- w443
    n184 = Negate(x=w437) -> (-x=w436:fxp<+/-,35,19>)
    n185 = Multiply(x=w443, y=w442) -> (x*y=w441:fxp<+/-,33,15>)
    n186 = Multiply(x=w436, y=w435) -> (x*y=w434:fxp<+/-,34,20>)
    n187 = Multiply(x=w440, y=w441) -> (x*y=→"Dyr_sin_d":fxp<+/-,33,15>)
    n188 = Multiply(x="Sin magnitude_y", y=w432) -> (x*y=w448:fxp<+/-,37,8>)
    n189 = Multiply(x=w432, y=w434) -> (x*y=→"Dyr_sin_dd":fxp<+/-,35,20>)
    n190 = Add(x=w448, y="Sin offset_y") -> (x+y=→"Dyr_sin":fxp<+/-,37,8>)
    n191 = local read "Sin wave freq._p (Hz)"() -> (w409:fxp<+/-,32,6>)
    n192 = local read "Time now(s)"() -> (w427:fxp<+,52,14>)
    n193 = local read "Sin magnitude_p"() -> (w410:fxp<+/-,21,6>)
    n194 = local read "Sin magnitude_p"() -> (w412:fxp<+/-,21,6>)
    n195 = local read "Sin omega_p"() -> (w411:fxp<+/-,34,9>)
    n196 = Multiply(x="Sin wave freq._p (Hz)", y=fxp<+/-,10,3> 2.0) -> (x*y=w431:fxp<+/-,42,9>)
    n197 = Multiply(x=w431, y=w427) -> (x*y=w428:fxp<+/-,41,19>)
    n198 = Square(x=w411) -> (x^2=w423:fxp<+,34,18>)
    n199 = xnode "High Throughput Sine & Cosine"("x (pi)"=w428) -> ("sin(x)"=w414:fxp<+/-,16,2>, "cos(x)"=w419:fxp<+/-,16,2>)
    n200 = Multiply(x=w413, y=w409) -> (x*y=w426:fxp<+/-,34,9>)
    "Sin omega_p" <- w426
    n201 = Negate(x=w423) -> (-x=w422:fxp<+/-,35,19>)
    n202 = Multiply(x=w426, y=w410) -> (x*y=w425:fxp<+/-,33,15>)
    n203 = Multiply(x=w422, y=w412) -> (x*y=w421:fxp<+/-,35,19>)
    n204 = Multiply(x=w419, y=w425) -> (x*y=→"Dpr_sin_d":fxp<+/-,33,15>)
    n205 = Multiply(x=w414, y=w421) -> (x*y=→"Dpr_sin_dd":fxp<+/-,35,20>)
    n206 = Multiply(x="Sin magnitude_p", y=w414) -> (x*y=w417:fxp<+/-,37,8>)
    n207 = Add(x=w417, y="Sin offset_p") -> (x+y=→"Dpr_sin":fxp<+/-,37,8>)
  }
  n208 = while "Time reset" {
    shift-right: [w524] -> _
    shift-left: _ -> [w525]
    shift-right: [w519] -> _
    shift-left: _ -> [w520]
    stop <- FALSE stop-if-true
    n209 = local read "Stop motor_y"() -> (w526:bool)
    n210 = call "Tick Count3"() -> ("Tick Count(uSec)"=w524:u32)
    n211 = Subtract(x=w524, y=w525) -> (x-y=w523:u32)
    n212 = Add(x=w520, y=w523) -> (x+y=w522:u32)
    n213 = Select(t=u32 0, s=w526, f=w522) -> (s? t:f=w519:u32)
    n214 = To Fixed-Point(number=w519) -> (fixed-point=w518:fxp<+,32,32>)  [unwired: 1 in]
    n215 = Multiply(x=fxp<+,20,-18> 1.0000003385357559e-06, y=w518) -> (x*y=→"Time now(s)":fxp<+,52,14>)
  }
  n216 = while "Ini" {
    stop <- FALSE stop-if-true
    n217 = case shown="True" "Ini coe." {
      frame False {
      }
      frame True {
        w544 = i16 0 items=["Step", "Sine"] ("Command_p")
        w545 = i16 2 items=["Raw", "Avg.", "Avg. w. filter"] ("Strain selection_p")
        w546 = i16 0 items=["Step", "Sine"] ("Command_y")
        w547 = i16 2 items=["Raw", "Avg.", "Avg. w. filter"] ("Strain selection_y")
        w549 = fxp<+/-,25,-10> -5.851034075021744e-07  # S/F coeff_p
        w548 = fxp<+/-,25,-10> -1.0477961041033268e-06  # S/F coeff_y
        w555 = i16 0 items=["Backward", "Forward"] ("Drive mode")
        n218 = local write "Sin wave freq._y (Hz)"(fxp<+/-,32,6> 1.0 ("Sin wave freq. (Hz)")) -> ()
        n219 = local write "Sin magnitude_y"(fxp<+/-,22,7> 5.0 ("Sin magnitude")) -> ()
        n220 = local write "fy_tolorance"(fxp<+,22,6> 5.0 ("f_tolorance")) -> ()
        n221 = local write "Sin offset_y"(fxp<+/-,38,9> 0.0 ("Sin offset")) -> ()
        n222 = local write "Dyr_step"(fxp<+/-,22,7> 0.0 ("Dr")) -> ()
        n223 = local write "Kp_y"(fxp<+/-,36,9> 30.0 ("Kp")) -> ()
        n224 = local write "Kd_y"(fxp<+/-,36,9> 0.0 ("Kd")) -> ()
        n225 = local write "Kv_y"(fxp<+/-,22,8> 0.0 ("Kv")) -> ()
        n226 = local write "Bv_y"(fxp<+/-,22,8> 0.0 ("Bv")) -> ()
        n227 = local write "Ki_y"(fxp<+/-,36,9> 0.0 ("Ki")) -> ()
        n228 = local write "S/F coeff_p"(w549) -> ()
        n229 = local write "S/F coeff_y"(w548) -> ()
        n230 = local write "dFy_add"(FALSE ("dF_add")) -> ()
        n231 = local write "dFp_add"(FALSE ("dFp_add")) -> ()
        n232 = local write "Sin wave freq._p (Hz)"(fxp<+/-,32,6> 1.0 ("Sin wave freq._p (Hz)")) -> ()
        n233 = local write "Sin magnitude_p"(fxp<+/-,21,6> 5.0 ("Sin magnitude_p")) -> ()
        n234 = local write "fp_tolorance"(fxp<+,22,6> 5.0 ("fp_tolorance")) -> ()
        n235 = local write "Sin offset_p"(fxp<+/-,22,7> 0.0 ("Sin offset_p")) -> ()
        n236 = local write "Dpr_step"(fxp<+/-,22,7> 0.0 ("Dpr_step")) -> ()
        n237 = local write "Kp_p"(fxp<+/-,36,9> 30.0 ("Kp_p")) -> ()
        n238 = local write "Kd_p"(fxp<+/-,36,9> 0.0 ("Kd_p")) -> ()
        n239 = local write "Kv_p"(fxp<+/-,22,8> 0.0 ("Kv_p")) -> ()
        n240 = local write "Bv_p"(fxp<+/-,22,8> 0.0 ("Bv_p")) -> ()
        n241 = local write "Ki_p"(fxp<+/-,36,9> 0.0 ("Ki_p")) -> ()
        n242 = local write "Strain selection_p"(w545) -> ()
        n243 = local write "Strain selection_y"(w547) -> ()
        n244 = local write "Command_p"(w544) -> ()
        n245 = local write "Command_y"(w546) -> ()
        n246 = local write "Drive mode"(w555) -> ()
        n247 = local write "Belt_mp"(fxp<+/-,6,6> 16.0 ("Belt_mp")) -> ()
        n248 = local write "Belt_my"(fxp<+/-,6,6> 16.0 ("Belt_my")) -> ()
        n249 = local write "Belt_op"(fxp<+/-,7,7> 22.0 ("Belt_op")) -> ()
        n250 = local write "Belt_oy"(fxp<+/-,7,7> 22.0 ("Belt_oy")) -> ()
      }
    }
  }
  n251 = while "FIFO" {
    stop <- FALSE stop-if-true
    n252 = flat-sequence {
      frame #0 {
        n253 = call "Loop Timer"("Count(uSec)"=u32 1000) -> ()  [unwired: 1 out]
      }
      frame #1 {
        n254 = local read "Strain_y (Avg8)"() -> (w579:fxp<+/-,36,4>)
        n255 = local read "Strain_y (Avg8 w. f)"() -> (w578:fxp<+/-,36,8>)
        n256 = local read "Dy_d (mm/s)"() -> (w575:fxp<+/-,36,11>)
        n257 = local read "Strain_y (Avg4 w. f)"() -> (w576:fxp<+/-,35,7>)
        n258 = local read "Strain_y (Avg2 w. f)"() -> (w564:fxp<+/-,34,7>)
        n259 = local read "D_p(mm)"() -> (w573:fxp<+/-,32,7>)
        n260 = local read "Raw Strain_p"() -> (w572:fxp<+/-,36,4>)
        n261 = local read "Strain_p (Avg8)"() -> (w571:fxp<+/-,36,4>)
        n262 = local read "Strain_p (Avg8 w. f)"() -> (w570:fxp<+/-,36,8>)
        n263 = local read "D_y(mm)"() -> (w581:fxp<+/-,32,7>)
        n264 = local read "Raw Strain_y"() -> (w580:fxp<+/-,36,4>)
        n265 = local read "Force_y"() -> (w574:fxp<+/-,32,10>)
        n266 = local read "Force_p"() -> (w569:fxp<+/-,32,10>)
        n267 = local read "Dp_d (mm/s)"() -> (w568:fxp<+/-,36,11>)
        n268 = local read "Fp_dc"() -> (w567:fxp<+/-,32,10>)
        n269 = Build Array(w581, w580, w579, w578, w574, w575, w576, w564, w573, w572, w571, w570, w569, w568, w567, fxp<+/-,40,8> 0.0 ("element")) -> (w565:fxp<+/-,43,11>[])
        n270 = xnode ("FIFO Write")("Element"=w565, "Timeout"=0) -> ()  [unwired: 1 in, 2 out]
      }
    }
  }
  n271 = while "PID force controller_y" {
    stop <- FALSE stop-if-true
    n272 = local read "Force_y"() -> (w599:fxp<+/-,32,10>)
    n273 = local read "fyt_d"() -> (w583:fxp<+/-,36,18>)
    n274 = local read "Fr_y"() -> (w585:fxp<+/-,32,10>)
    n275 = xnode "High Throughput Subtract"("x"=w585, "y"=w599) -> ("x-y"=w598:fxp<+/-,33,11>)
    "fy_tilde" <- w598
    n276 = Absolute Value(x=w598) -> (abs(x)=w589:fxp<+,33,11>)
    n277 = local read "fyt_i"() -> (w584:fxp<+/-,36,16>)
    n278 = xnode ("High Throughput Multiply")("x"="Kp_y", "y"=w598) -> ("x*y"=w596:fxp<+/-,64,20>)
    n279 = xnode ("High Throughput Multiply")("x"="Kd_y", "y"=w583) -> ("x*y"=w595:fxp<+/-,64,27>)
    n280 = xnode ("High Throughput Add")("x"=w596, "y"=w595) -> ("x+y"=w592:fxp<+/-,64,28>)
    n281 = xnode ("High Throughput Multiply")("x"="Ki_y", "y"=w584) -> ("x*y"=w593:fxp<+/-,64,25>)
    n282 = Greater?(x=w589, y="fy_tolorance") -> (0:w587:bool)
    n283 = xnode ("High Throughput Add")("x"=w592, "y"=w593) -> ("x+y"=w591:fxp<+/-,64,29>)
    n284 = Select(t=w591, s=w587, f=fxp<+/-,51,14> 0.0) -> (s? t:f=→"Fy_PID":fxp<+/-,64,29>)
  }
  n285 = while "Quadrature drive_p" {
    stop <- FALSE stop-if-true
    n286 = local read "dFp_PID"() -> (w602:fxp<+/-,36,18>)
    n287 = local read "omega_p (rad/s)"() -> (w608:fxp<+/-,20,9>)
    n288 = local read "Fp_PID"() -> (w603:fxp<+/-,36,16>)
    n289 = Select(t=w602, s="dFp_add", f=fxp<+,1,1> 0.0) -> (s? t:f=w606:fxp<+/-,36,18>)
    n290 = call "Oriental_step_motor_PKP225.vi"("F_Threshold"=fxp<+,12,12> 10.0, "dFmr"=w606, "omega"=w608, "Fmr"=w603) -> ("vq_F"=→"vq_p_F":fxp<+/-,20,5>, "vd_F"=→"vd_p_F":fxp<+/-,20,5>)  [unwired: 6 in]
  }
  n291 = while "PID force controller_p" {
    stop <- FALSE stop-if-true
    n292 = local read "Force_p"() -> (w623:fxp<+/-,32,10>)
    n293 = local read "fpt_d"() -> (w614:fxp<+/-,36,18>)
    n294 = local read "Fr_p"() -> (w624:fxp<+/-,32,10>)
    n295 = xnode "High Throughput Subtract"("x"=w624, "y"=w623) -> ("x-y"=w615:fxp<+/-,33,11>)
    "fp_tilde" <- w615
    n296 = local read "fpt_i"() -> (w612:fxp<+/-,34,18>)
    n297 = xnode ("High Throughput Multiply")("x"="Kp_p", "y"=w615) -> ("x*y"=w613:fxp<+/-,64,20>)
    n298 = xnode ("High Throughput Multiply")("x"="Kd_p", "y"=w614) -> ("x*y"=w629:fxp<+/-,64,27>)
    n299 = Absolute Value(x=w615) -> (abs(x)=w622:fxp<+,33,11>)
    n300 = xnode ("High Throughput Add")("x"=w613, "y"=w629) -> ("x+y"=w627:fxp<+/-,64,28>)
    n301 = xnode ("High Throughput Multiply")("x"="Ki_p", "y"=w612) -> ("x*y"=w628:fxp<+/-,64,27>)
    n302 = xnode ("High Throughput Add")("x"=w627, "y"=w628) -> ("x+y"=w618:fxp<+/-,64,29>)
    n303 = Greater?(x=w622, y="fp_tolorance") -> (0:w619:bool)
    n304 = Select(t=w618, s=w619, f=fxp<+,1,1> 0.0) -> (s? t:f=→"Fp_PID":fxp<+/-,64,29>)
  }
  n305 = while "PD position controller_p" {
    stop <- FALSE stop-if-true
    n306 = local read "Drive mode"() -> (w632:i16)
    n307 = case shown="0, Default" w632 {
      tunnel: [fxp<+/-,62,19> 0.0 w635] -> w631
      frame 0, Default {
        # "Backward"
      }
      frame 1 {
        # "Forward"
        n308 = local read "D_p(mm)"() -> (w642:fxp<+/-,32,7>)
        n309 = local read "Dp_error_d"() -> (w634:fxp<+/-,33,8>)
        n310 = local read "Dpr_for"() -> (w641:fxp<+/-,22,7>)
        n311 = Subtract(x=w641, y=w642) -> (x-y=w640:fxp<+/-,24,8>)
        "Dp_error" <- w640
        n312 = Multiply(x=w640, y="Kv_p") -> (x*y=w637:fxp<+/-,34,16>)
        n313 = Multiply(x=w634, y="Bv_p") -> (x*y=w636:fxp<+/-,55,16>)
        n314 = Add(x=w637, y=w636) -> (x+y=w635:fxp<+/-,56,17>)
      }
    }
    "Fr_p" <- w631
  }
  n315 = while "All switch" {
    stop <- FALSE stop-if-true
    n316 = case shown="False" "Encoder reset" {
      frame False {
        n317 = local write "Encoder reset_p"(FALSE ("Encoder reset_p")) -> ()
        n318 = local write "Encoder reset_y"(FALSE ("Encoder reset_y")) -> ()
      }
      frame True {
        n319 = local write "Encoder reset_p"(TRUE ("Encoder reset_p")) -> ()
        n320 = local write "Encoder reset_y"(TRUE ("Encoder reset_y")) -> ()
      }
    }
  }
  n321 = while "Derivative" {
    stop <- FALSE stop-if-true
    n322 = local read "Dpr_sin_dd"() -> (w657:fxp<+/-,35,20>)
    n323 = local read "Stop motor_y"() -> (w663:bool)
    n324 = local read "Dyr_sin_dd"() -> (w665:fxp<+/-,35,20>)
    n325 = local read "Dpr_sin_d"() -> (w659:fxp<+/-,33,15>)
    n326 = local read "Stop motor_p"() -> (w655:bool)
    n327 = local read "Dyr_sin_d"() -> (w668:fxp<+/-,33,15>)
    n328 = local read "Dp_error"() -> (w660:fxp<+/-,22,7>)
    n329 = local read "Dy_error"() -> (w669:fxp<+/-,22,7>)
    n330 = local read "Dp_dd"() -> (w658:fxp<+/-,36,25>)
    n331 = local read "Dy_dd"() -> (w666:fxp<+/-,36,25>)
    n332 = Subtract(x=w668, y=w669) -> (x-y=w667:fxp<+/-,34,16>)
    n333 = Subtract(x=w665, y=w666) -> (x-y=w664:fxp<+/-,41,26>)
    n334 = Subtract(x=w659, y=w660) -> (x-y=w652:fxp<+/-,34,16>)
    n335 = Subtract(x=w657, y=w658) -> (x-y=w656:fxp<+/-,41,26>)
    n336 = Select(t=fxp<+,1,1> 0.0, s=w663, f=w667) -> (s? t:f=→"Dy_error_d":fxp<+/-,34,16>)
    n337 = Select(t=fxp<+/-,64,49> 0.0, s=w663, f=w664) -> (s? t:f=→"Dy_error_dd":fxp<+/-,64,49>)
    n338 = Select(t=fxp<+,1,1> 0.0, s=w655, f=w652) -> (s? t:f=→"Dp_error_d":fxp<+/-,34,16>)
    n339 = Select(t=fxp<+/-,41,26> 0.0, s=w655, f=w656) -> (s? t:f=→"Dp_error_dd":fxp<+/-,41,26>)
  }
  n340 = while "ft_d" {
    stop <- FALSE stop-if-true
    n341 = local read "Dy_error_dd"() -> (w687:fxp<+/-,36,16>)
    n342 = local read "Dp_error_dd"() -> (w678:fxp<+/-,36,16>)
    n343 = local read "Dy_error_d"() -> (w689:fxp<+/-,33,8>)
    n344 = local read "Dp_error_d"() -> (w680:fxp<+/-,33,8>)
    n345 = local read "Kv_p"() -> (w681:fxp<+/-,22,8>)
    n346 = local read "Bv_p"() -> (w679:fxp<+/-,22,8>)
    n347 = local read "Kv_y"() -> (w690:fxp<+/-,22,8>)
    n348 = local read "Bv_y"() -> (w688:fxp<+/-,22,8>)
    n349 = local read "Force_y"() -> (w683:fxp<+/-,32,10>)
    n350 = Multiply(x=w689, y=w690) -> (x*y=w685:fxp<+/-,55,16>)
    n351 = Multiply(x=w687, y=w688) -> (x*y=w686:fxp<+/-,58,24>)
    n352 = Multiply(x=w680, y=w681) -> (x*y=w676:fxp<+/-,55,16>)
    n353 = Multiply(x=w678, y=w679) -> (x*y=w677:fxp<+/-,58,24>)
    n354 = local read "Force_p"() -> (w674:fxp<+/-,32,10>)
    n355 = Add(x=w685, y=w686) -> (x+y=w684:fxp<+/-,63,24>)
    n356 = Add(x=w676, y=w677) -> (x+y=w675:fxp<+/-,63,24>)
    n357 = Subtract(x=w684, y=w683) -> (x-y=→"fyt_d":fxp<+/-,63,24>)
    n358 = Subtract(x=w675, y=w674) -> (x-y=→"fpt_d":fxp<+/-,63,24>)
  }
  n359 = while "Encoder_p" {
    shift-right: [w705] -> _
    shift-left: _ -> [w706]
    shift-right: [w707] -> _
    shift-left: _ -> [w708]
    shift-right: [w701] -> _
    shift-left: _ -> [w709]
    stop <- FALSE stop-if-true
    w695 = fxp<+/-,20,-5> 0.002499997615814209  # L/800
    n360 = xnode "FPGA I/O Node"() -> ("Mod4/DI0"=w703:bool, "Mod4/DI1"=w704:bool)  [unwired: 2 in, 2 out]
    n361 = local read "Belt_mp"() -> (w694:fxp<+/-,6,6>)
    n362 = local read "Belt_op"() -> (w692:fxp<+/-,7,7>)
    n363 = call "encoder_sub.vi"("A_pre"=w706, "B_pre"=w708, "Encoder Position_pre"=w709, "A input"=w703, "Encoder Position Reset"="Encoder reset_p", "B input"=w704) -> ("A"=w705:bool, "B"=w707:bool, "Encoder Position (Counts)"=w701:i32)  [unwired: 19 in]
    "Encoder Position_p" <- w701
    n364 = Multiply(x=w695, y=w694) -> (x*y=w693:fxp<+/-,26,1>)
    n365 = To Fixed-Point(number=w701) -> (fixed-point=w700:fxp<+/-,32,32>)  [unwired: 1 in]
    n366 = Divide(x=w693, y=w692) -> (x/y=w691:fxp<+/-,33,1>)
    n367 = xnode ("High Throughput Multiply")("x"=w700, "y"=fxp<+/-,16,1> 0.125) -> ("x*y"=→"rad_p(NrTheta)":fxp<+/-,48,33>)
    n368 = xnode ("High Throughput Multiply")("x"=w700, "y"=w691) -> ("x*y"=→"D_p(mm)":fxp<+/-,64,33>)
  }
  n369 = while "Omega_p(T method)" {
    shift-right: [w725] -> _
    shift-left: _ -> [w723]
    shift-right: [w718] -> _
    shift-left: _ -> [w724]
    shift-right: [w720] -> _
    shift-left: _ -> [w722]
    stop <- FALSE stop-if-true
    w714 = fxp<+/-,32,0> 0.3183098859153688  # L/2/pi
    n370 = local read "Encoder Position_p"() -> (w725:i32)
    n371 = call "Tick Count4"() -> ("Tick Count(Ticks)"=w721:u32)
    n372 = call "omega_sub_Encoder_800ppr.vi"("mt0"="mt0_omega_p", "omega_pre"=w724, "ticks_m_pre"=w722, "ticks"=w721, "count_pre"=w723, "count"=w725) -> ("ticks_m"=w720:u32, "mt"=→"mt_omega_p":u32, "omega"=w718:fxp<+/-,20,9>)  [unwired: 3 in]
    "omega_p (rad/s)" <- w718
    n373 = Multiply(x=w714, y="Belt_mp") -> (x*y=w712:fxp<+/-,38,6>)
    n374 = Divide(x=w712, y="Belt_op") -> (x/y=w710:fxp<+/-,20,1>)
    n375 = xnode ("High Throughput Multiply")("x"=w710, "y"=w718) -> ("x*y"=→"Dp_d (mm/s)":fxp<+/-,40,10>)
  }
  n376 = xnode "FPGA I/O Node"("error in"=w1, "Mod6/Stop"=TRUE) -> ()  [unwired: 1 in, 2 out]
